vi "get_data.vi"(8 "error in (no error)":errorcluster, 11 "Counter in":refnum<class "Counter.lvclass">) -> (0 "error out":errorcluster, 3 "Counter out":refnum<class "Counter.lvclass">)   [LabVIEW 2013, in "Counter.lvclass"]
uses:
  Counter.lvclass
  Counter.lvclass/Counter.ctl
  <vilib>/DAQmx/read.llb/DAQmx Read (Counter 1D U32 1Chan NSamp).vi
  Experiment/Globals.vi
  <vilib>/DAQmx/miscellaneous.llb/DAQmx Fill In Error Info.vi
  Experiment/Experiment.lvclass
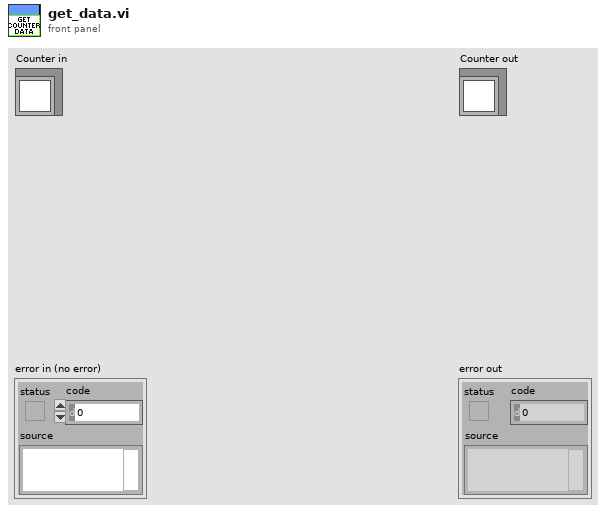
[diagram p1: front panel]
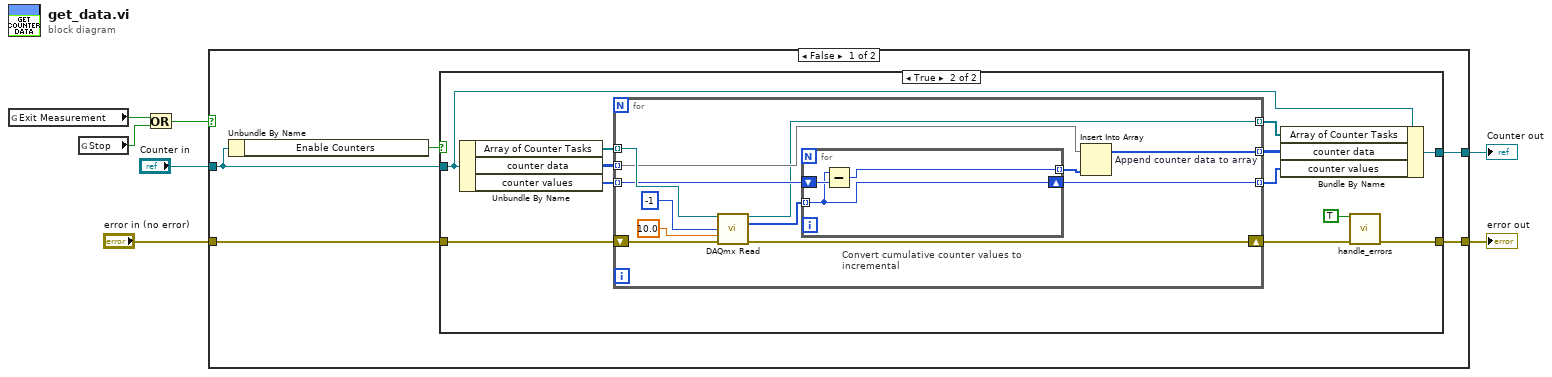
[diagram p0: block diagram]
diagram:
  n1 = global read "Globals.vi" "Exit Measurement"() -> (w4:bool)
  n2 = global read "Globals.vi" "Stop"() -> (w3:bool)
  n3 = Or(x=w4, y=w3) -> (x .or. y?=w2:bool)
  n4 = case shown="False" w2 {
    tunnel: [w8 w42] -> w5
    tunnel: [w11 w43] -> w6
    tunnel: "Counter in" -> [w10 w43]
    tunnel: "error in (no error)" -> [w9 w42]
    frame False {
      n5 = Unbundle By Name(w10) -> ("Enable Counters"=w12:bool)
      n6 = case shown="True" w12 {
        tunnel: w9 -> [w14 w26]
        tunnel: [w14 w15] -> w8
        tunnel: [w13 w25] -> w11
        tunnel: w10 -> [w13 w19]
        frame False {
        }
        frame True {
          n7 = Unbundle By Name(w19) -> ("Array of Counter Tasks"=w22:refnum<k21>[], "counter data"=w21:u32[][], "counter values"=w20:u32[])
          n8 = for {
            tunnel: w22 -> [w38] mode=indexing
            shift-right: [w36] -> w16
            shift-left: w26 -> [w37]
            tunnel: [w35] -> w23 mode=indexing
            tunnel: w21 -> [w34] mode=indexing
            tunnel: w20 -> [w33] mode=indexing
            tunnel: [w32] -> w18 mode=indexing
            tunnel: [w31] -> w24 mode=indexing
            n9 = call-poly <vilib>:"DAQmx Read.vi"("task/channels in"=w38, "number of samples per channel"=-1, "timeout"=10.0, "error in"=w37) -> ("task out"=w31:refnum<k21>, "data"=w28:u32[], "error out"=w36:errorcluster)  [unwired: 9 out]
            n10 = for "Convert cumulative counter values to incremental" {
              tunnel: w28 -> [w39] mode=indexing
              shift-right: [w39] -> w35
              shift-left: w33 -> [w41]
              tunnel: [w40] -> w27 mode=indexing
              n11 = Subtract(x=w39, y=w41) -> (x-y=w40:u32)
            }
            n12 = Insert Into Array "Append counter data to array"(array=w34, new element=w27) -> (w32:u32[])  [unwired: 1 in]
          }
          n13 = Bundle By Name(cluster=w19, "Array of Counter Tasks"=w24, "counter data"=w18, "counter values"=w23) -> (w25:refnum<class "Counter.lvclass">)
          n14 = call "handle_errors.vi"("Exit Operation"=TRUE ("Exit Measurement"), "error in (no error)"=w16) -> ("error out"=w15:errorcluster)  [unwired: 13 in]
        }
      }
    }
    frame True {
    }
  }
  "error out" <- w5
  "Counter out" <- w6
